vi "INIT.vi"(8 "error in (no error)":errorcluster, 11 "VIS-NIR_STRESING_NEW in":refnum<class "VIS-NIR_STRESING_NEW.lvclass">) -> (0 "error out":errorcluster, 3 "VIS-NIR_STRESING_NEW out":refnum<class "VIS-NIR_STRESING_NEW.lvclass">)   [LabVIEW 2020, in "VIS-NIR_STRESING_NEW.lvclass"]
uses:
  VIS-NIR_STRESING_NEW/VIS-NIR_STRESING_NEW.lvclass
  C:/dev/TRANCON/Classes/GeneralFunctionality/GeneralFunctionality.lvclass
  C:/dev/TRANCON/Classes/Detector/Detector.lvclass
  GeneralFunctionality/GeneralFunctionality.lvclass/GeneralFunctionality.ctl
  Config/Config.lvclass
  Detector.lvclass
  GeneralFunctionality/GeneralFunctionality.lvclass
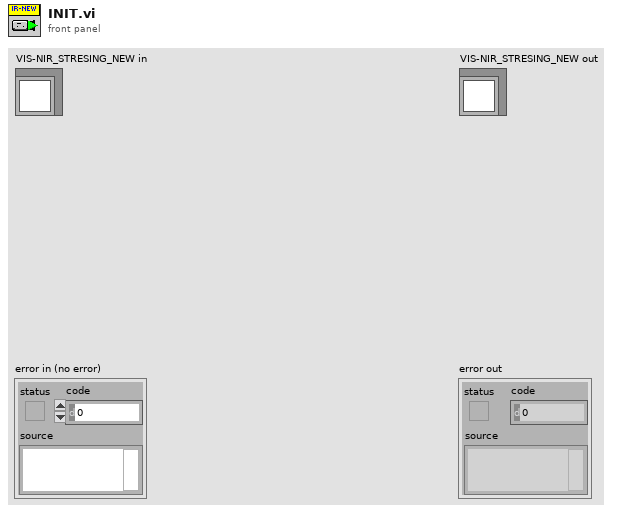
[diagram p1: front panel]
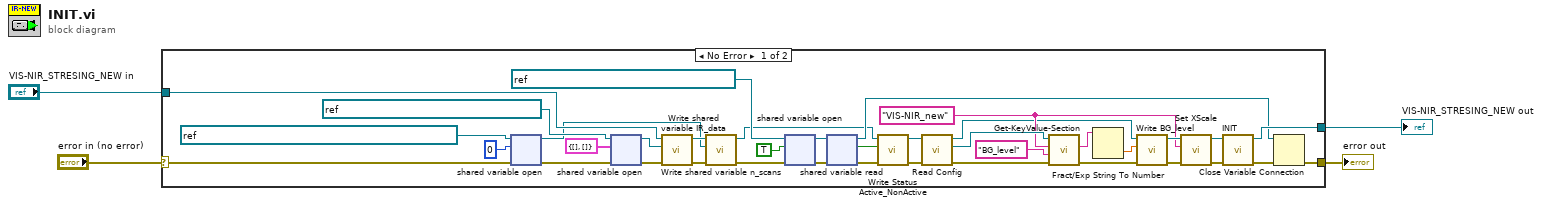
[diagram p0: block diagram]
diagram:
  n1 = case shown="No Error" "error in (no error)" {
    selector: "error in (no error)" -> [w11 w44]
    tunnel: "VIS-NIR_STRESING_NEW in" -> [w16 w43]
    tunnel: [w8 w44] -> w2
    tunnel: [w36 w43] -> w1
    frame No Error {
      w27 = "VIS-NIR_new" ("Section")
      n2 = shared-variable-open(refnum<k21> "ni.var.psp://localhost/IR_TRANCON/n_scans_IR" ("shared variable refnum in"), w11, 0) -> (w13:refnum<k21>, w18:errorcluster)  [unwired: 1 in]
      n3 = shared-variable-open(refnum<k21> "ni.var.psp://localhost/Lib_IR/IR_data" ("shared variable refnum in"), w18, cluster{"I":i32[][], "II":i32[][]} {"I"=[], "II"=[]} ("data out")) -> (w12:refnum<k21>, w10:errorcluster)  [unwired: 1 in]
      n4 = call-dynamic "Write shared variable IR_data.vi"("error in (no error)"=w10, "shared variable IR_data"=w12, "VIS-NIR_STRESING_NEW in"=w16) -> ("error out"=w17:errorcluster, "VIS-NIR_STRESING_NEW out"=w14:refnum<class "VIS-NIR_STRESING_NEW.lvclass">)  [unwired: 7 in]
      n5 = call-dynamic "Write shared variable n_scans.vi"("error in (no error)"=w17, "shared variable n_scans"=w13, "VIS-NIR_STRESING_NEW in"=w14) -> ("error out"=w9:errorcluster, "VIS-NIR_STRESING_NEW out"=w15:refnum<class "VIS-NIR_STRESING_NEW.lvclass">)  [unwired: 7 in]
      n6 = shared-variable-open(refnum<k21> "ni.var.psp://localhost/Lib_IR/working" ("shared variable refnum in"), w9, TRUE) -> (w40:refnum<k21>, w39:errorcluster)  [unwired: 1 in]
      n7 = shared-variable-read(w40, w39) -> (w23:refnum<k21>, w42:errorcluster, w41:bool)  [unwired: 1 out]
      n8 = call "Write Status Active_NonActive.vi"("error in (no error)"=w42, "Status Active/NonActive"=w41, "GeneralFunctionality in"=w15) -> ("error out"=w6:errorcluster, "GeneralFunctionality out"=w7:refnum<class "VIS-NIR_STRESING_NEW.lvclass">)  [unwired: 7 in]
      n9 = call "Read Config.vi"("error in (no error)"=w6, "GeneralFunctionality en entrée"=w7) -> ("error out"=w32:errorcluster, "Config.lvclass"=w33:refnum<class "Config.lvclass">, "GeneralFunctionality en sortie"=w5:refnum<class "VIS-NIR_STRESING_NEW.lvclass">)  [unwired: 7 in]
      n10 = call-dynamic "Get-KeyValue-Section.vi"("error in (no error)"=w32, "Key"="BG_level", "Section"=w27, "Config in"=w33) -> ("error out"=w29:errorcluster, "Value"=w30:string)  [unwired: 5 in, 1 out]
      n11 = Fract/Exp String To Number(string=w30) -> (number=w31:dbl)  [unwired: 3 in, 1 out]
      n12 = call-dynamic "Write BG_level.vi"("error in (no error)"=w29, "BG_level"=w31, "Detector in"=w5) -> ("error out"=w35:errorcluster, "Detector out"=w34:refnum<class "VIS-NIR_STRESING_NEW.lvclass">)  [unwired: 7 in]
      n13 = call "Set XScale.vi"("error in (no error)"=w35, "Section"=w27, "Detector en entrée"=w34) -> ("error out"=w24:errorcluster, "Detector en sortie"=w26:refnum<class "VIS-NIR_STRESING_NEW.lvclass">)  [unwired: 7 in]
      n14 = call-parent "INIT.vi"("error in (no error)"=w24, "Detector in"=w26) -> ("error out"=w25:errorcluster, "Detector out"=w36:refnum<class "VIS-NIR_STRESING_NEW.lvclass">)  [unwired: 8 in]
      n15 = Close Variable Connection(8:w25, 11:w23) -> (0:w8:errorcluster)
    }
    frame Error {
    }
  }
  "error out" <- w2
  "VIS-NIR_STRESING_NEW out" <- w1
